vi "CODcr启动命令.vi"(11 "输入参数":T1) -> ()   [LabVIEW 2016, in "CODCr库.lvlib"]
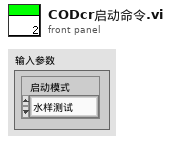
[diagram p1: front panel]
types:
  T1 = cluster{"启动模式":enum16{"水样测试", "空白核查", "跨度核查", "校零", "校标"}}
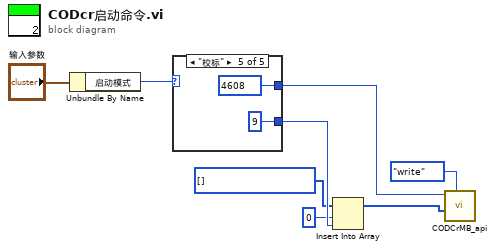
[diagram p0: block diagram]
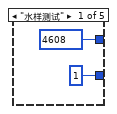
[diagram p2: hidden frame]
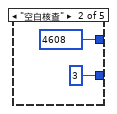
[diagram p3: hidden frame]
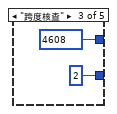
[diagram p4: hidden frame]
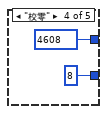
[diagram p5: hidden frame]
diagram:
  n1 = Unbundle By Name("输入参数") -> ("启动模式"=w4:enum16{"水样测试", "空白核查", "跨度核查", "校零", "校标"})
  n2 = case shown="\"校标\"" w4 {
    tunnel: [u16 4608 ("address") u16 4608 ("address") u16 4608 ("address") u16 4608 ("address") u16 4608 ("address")] -> w2
    tunnel: [u16 1 ("address") u16 3 ("address") u16 2 ("address") u16 8 ("address") u16 9 ("address")] -> w7
    frame "水样测试" {
    }
    frame "空白核查" {
    }
    frame "跨度核查" {
    }
    frame "校零" {
    }
    frame "校标" {
    }
  }
  n3 = Insert Into Array(array=u16[] [] ("values"), index=0 ("索引"), new element=w7) -> (w1:u16[])
  n4 = call "CODCrMB_api.vi"("STEP"=enum16{"open", "read", "write", "close"}."write", "values"=w1, "starting address"=w2) -> ()  [unwired: 6 in, 3 out]
